vi "Module Loop.vi"(8 "error in (no error)":errorcluster, 11 "Messaging Client in":refnum<class "Messaging Server Client.lvclass">) -> (0 "error out":errorcluster, 3 "Messaging Client out":refnum<class "Messaging Server Client.lvclass">)   [LabVIEW 2020, in "Volatus.lvlib" / "Messaging Server Client.lvclass"]
uses:
  Messaging Server Client.lvclass
  Messaging Server Client.lvclass/Messaging Server Client.ctl
  Module/Module.lvclass
  lv-vecto/Vecto/proto/ConnectStatus/Enumeration.ctl
  lv-vecto/Vecto/proto/ConnectStatus/ConnectStatus.lvlib
  C:/dev/lv20CE/relink/lv-volatus/Volatus/Module/Module.lvclass
  C:/dev/lv20CE/relink/lv-volatus/Volatus/Messaging Client/Messaging Server Client.lvclass
  Event Level.ctl
  Volatus.lvlib
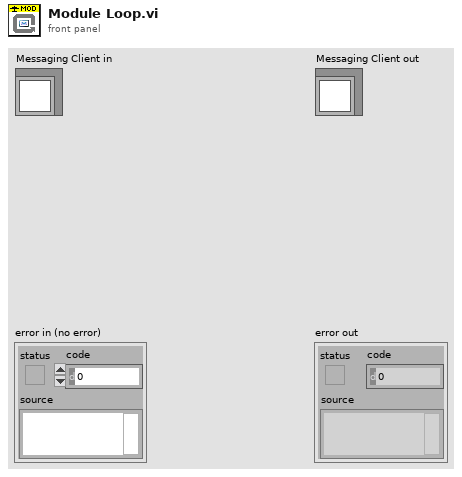
[diagram p1: front panel]
types:
  T1 = enum32{"Invalid", "Standard", "Closed", "Hidden", "Minimized", "Maximized"}
  T2 = typedef "Volatus.lvlib/Event Level.ctl" = enum16{"Debug", "Info", "Warning", "Error"}
  T3 = typedef "ConnectStatus.lvlib/Enumeration.ctl" = enum16{"STATUS_UNKNOWN", "STATUS_SUCCESS", "STATUS_ERROR", "STATUS_BAD_CONFIG", "STATUS_BAD_SYSTEM", "STATUS_BAD_CLUSTER", "STATUS_NOT_ALLOWED"}
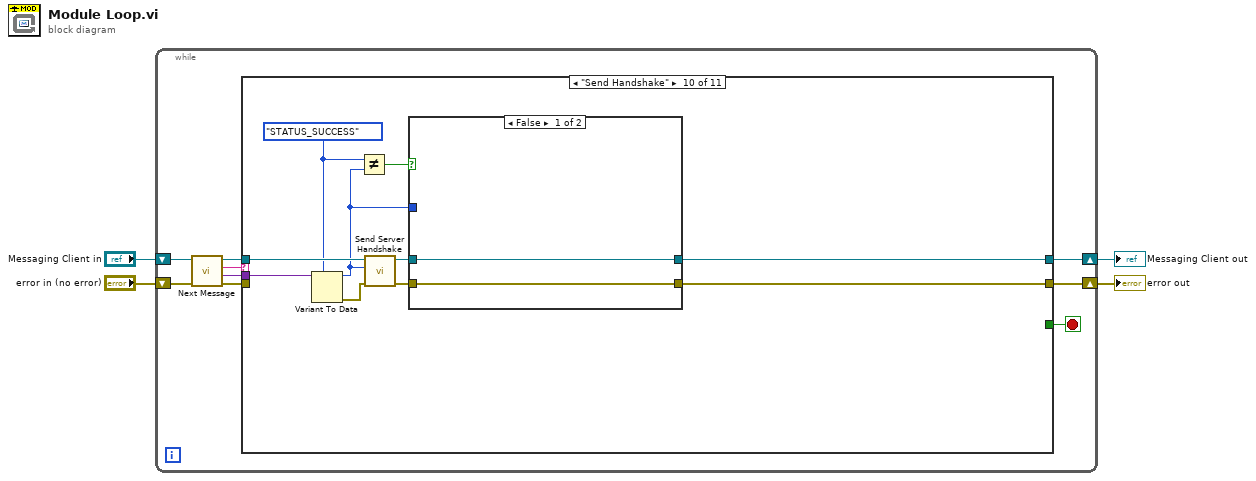
[diagram p0: block diagram]
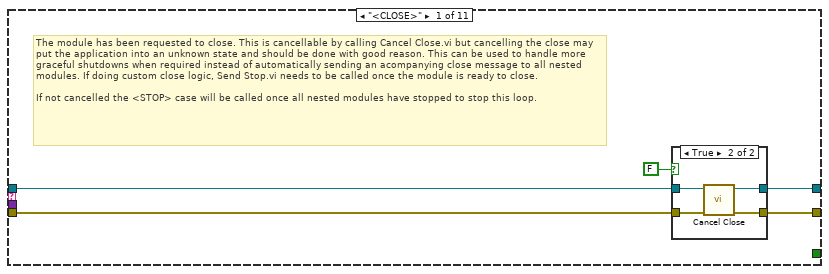
[diagram p2: hidden frame]
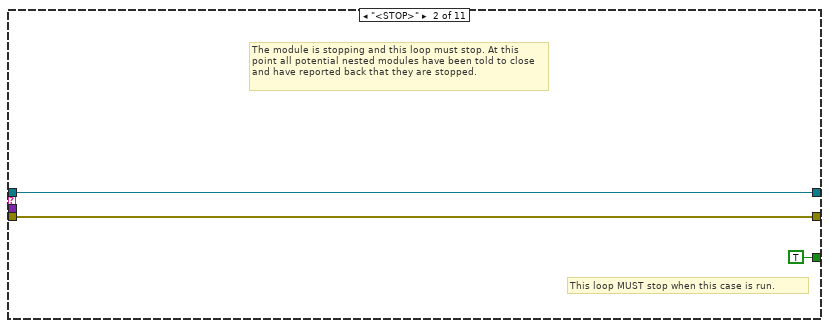
[diagram p4: hidden frame]
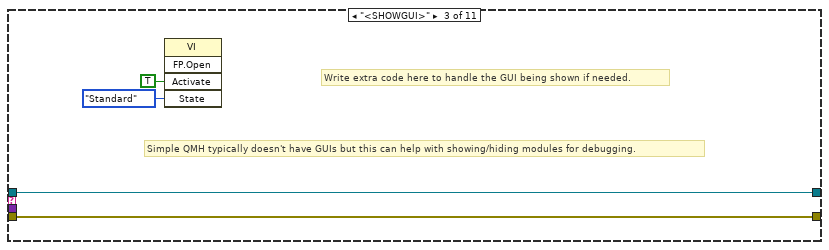
[diagram p5: hidden frame]
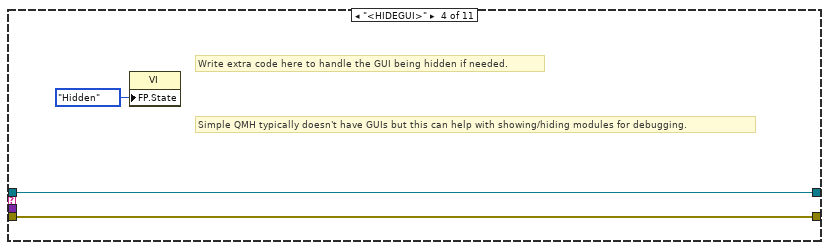
[diagram p6: hidden frame]
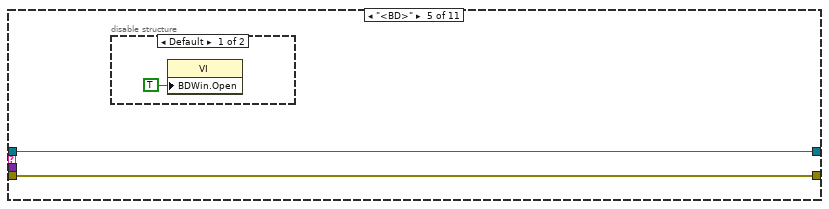
[diagram p7: hidden frame]
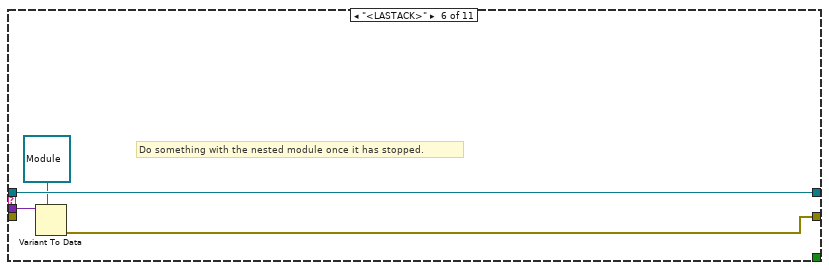
[diagram p9: hidden frame]
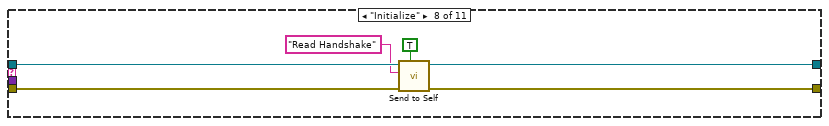
[diagram p11: hidden frame]
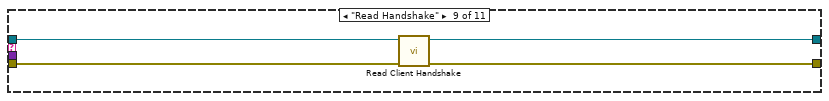
[diagram p12: hidden frame]
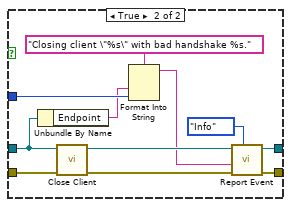
[diagram p13: hidden frame]
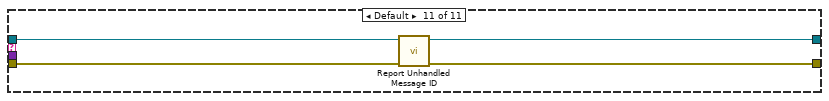
[diagram p14: hidden frame]
diagram:
  n1 = while {
    shift-right: [w8] -> w2
    shift-left: "Messaging Client in" -> [w13]
    shift-right: [w7] -> w1
    shift-left: "error in (no error)" -> [w12]
    stop <- w6 stop-if-true
    n2 = call "Next Message.vi"("error in (no error)"=w12, "Module in"=w13) -> ("error out"=w11:errorcluster, "Data"=w5:variant, "ID"=w10:string, "Module out"=w9:refnum<class "Messaging Server Client.lvclass">)  [unwired: 6 in]
    n3 = case shown="\"Send Handshake\"" w10 {
      tunnel: w11 -> [w14 w26 w30 w33 w35 _ w42 w49 w53 _ w80]
      tunnel: w9 -> [w15 w27 w31 w34 w36 w41 w43 w47 w51 w62 w78]
      tunnel: [w17 w27 w31 w34 w36 w41 w43 w46 w50 w56 w77] -> w8
      tunnel: [w18 w26 w30 w33 w35 w38 w42 w48 w52 w55 w79] -> w7
      tunnel: [_ TRUE _ _ _ _ _ _ _ _ _] -> w6
      tunnel: w5 -> [_ _ _ _ _ w40 _ _ _ w63 _]
      frame "<CLOSE>" {
        # "The module has been requested to close. This is cancellable by calling Cancel Close.vi but cancelling the close may put the application into an unknown state and should be done with good reason. This can be used to handle more graceful shutdowns when required instead of automatically sending an acompanying close message to all nested modules. If doing custom close logic, Send Stop.vi needs to be called once the module is ready to close.\n\nIf not cancelled the <STOP> case will be called once all nested modules have stopped to stop this loop."
        n4 = case shown="True" FALSE {
          tunnel: w14 -> [w19 w24]
          tunnel: [w19 w23] -> w18
          tunnel: w15 -> [w20 w22]
          tunnel: [w20 w21] -> w17
          frame False {
          }
          frame True {
            n5 = call "Cancel Close.vi"("error in (no error)"=w24, "Module in"=w22) -> ("error out"=w23:errorcluster, "Module out"=w21:refnum<class "Messaging Server Client.lvclass">)  [unwired: 8 in]
          }
        }
      }
      frame "<STOP>" {
        # "This loop MUST stop when this case is run."
        # "The module is stopping and this loop must stop. At this point all potential nested modules have been told to close and have reported back that they are stopped."
      }
      frame "<SHOWGUI>" {
        # "Simple QMH typically doesn't have GUIs but this can help with showing/hiding modules for debugging."
        # "Write extra code here to handle the GUI being shown if needed."
        n6 = invoke class="VI" method="FP.Open"("Activate"=TRUE ("Activate?"), "State"=T1."Standard") -> ()  [unwired: 3 in, 5 out]
      }
      frame "<HIDEGUI>" {
        # "Simple QMH typically doesn't have GUIs but this can help with showing/hiding modules for debugging."
        # "Write extra code here to handle the GUI being hidden if needed."
        n7 = property class="VI"("FP.State"=T1."Hidden" ("Front Panel Window:State")) -> ()  [unwired: 2 in, 2 out]
      }
      frame "<BD>" {
        n8 = disable-structure shown="Default" {
          frame condition #0 (active) {
            n9 = property class="VI"("BDWin.Open"=TRUE ("Block Diagram Window:Open")) -> ()  [unwired: 2 in, 2 out]
          }
          frame condition #1 {
          }
        }
      }
      frame "<LASTACK>" {
        # "Do something with the nested module once it has stopped."
        n10 = Variant To Data(type=refnum<class "Module.lvclass"> refnum ("Volatus:Module"), Variant=w40) -> (error out=w38:errorcluster)  [unwired: 1 in, 1 out]
      }
      frame "<TIMEOUT>" {
      }
      frame "Initialize" {
        n11 = call "Send to Self.vi"("High Priority (F)"=TRUE, "error in (no error)"=w49, "Message ID"="Read Handshake", "Module in"=w47) -> ("error out"=w48:errorcluster, "Module out"=w46:refnum<class "Messaging Server Client.lvclass">)  [unwired: 6 in]
      }
      frame "Read Handshake" {
        n12 = call "Read Client Handshake.vi"("error in (no error)"=w53, "Messaging Server Client in"=w51) -> ("error out"=w52:errorcluster, "Messaging Server Client out"=w50:refnum<class "Messaging Server Client.lvclass">)  [unwired: 8 in]
      }
      frame "Send Handshake" {
        w60 = Enumeration."STATUS_SUCCESS" ("Handshake Status")
        n13 = Variant To Data(type=w60, Variant=w63) -> (data=w54:T3, error out=w61:errorcluster)  [unwired: 1 in]
        n14 = Not Equal?(x=w60, y=w54) -> (x != y?=w57:bool)
        n15 = call "Send Server Handshake.vi"("error in (no error)"=w61, "Enumeration"=w54, "Messaging Client in"=w62) -> ("error out"=w59:errorcluster, "Messaging Client out"=w58:refnum<class "Messaging Server Client.lvclass">)  [unwired: 7 in]
        n16 = case shown="False" w57 {
          tunnel: w59 -> [w64 w76]
          tunnel: w58 -> [w65 w73]
          tunnel: [w65 w68] -> w56
          tunnel: [w64 w70] -> w55
          tunnel: w54 -> [_ w74]
          frame False {
          }
          frame True {
            n17 = Unbundle By Name(w73) -> ("Endpoint"=w72:string)
            n18 = call "Close Client.vi"("error in (no error)"=w76, "Messaging Server Client in"=w73) -> ("error out"=w75:errorcluster, "Messaging Server Client out"=w69:refnum<class "Messaging Server Client.lvclass">)  [unwired: 8 in]
            n19 = Format Into String(format string="Closing client \"%s\" with bad handshake %s.", w72, w74) -> (resulting string=w67:string)  [unwired: 2 in, 1 out]
            n20 = call "Report Event.vi"("Level (Info)"=Event_Level."Info", "error in (no error)"=w75, "Message"=w67, "Module in"=w69) -> ("error out"=w70:errorcluster, "Module out"=w68:refnum<class "Messaging Server Client.lvclass">)  [unwired: 6 in]
          }
        }
      }
      frame Default {
        n21 = call "Report Unhandled Message ID.vi"("error in (no error)"=w80, "Module in"=w78) -> ("error out"=w79:errorcluster, "Module out"=w77:refnum<class "Messaging Server Client.lvclass">)  [unwired: 8 in]
      }
    }
  }
  "error out" <- w1
  "Messaging Client out" <- w2
